vi "Pre Launch Init.vi"(11 "AsmTestMachine in":refnum<class "AsmTestMachine.lvclass">) -> (0 "error out":errorcluster, 3 "AsmTestMachine out":refnum<class "AsmTestMachine.lvclass">)   [LabVIEW 2021, in "AsmTestMachine.lvlib" / "AsmTestMachine.lvclass"]
doc: "(<B>Filename</B>: Actor Framework.lvlib:Actor.lvclass:Pre Launch Init.vi)\n\nDefines behavior that occurs after the Launch Nested Actor method is invoked but before the actor's Actor Core method begins running.\n\nBy default, this method does nothing. A descendant class may override it to define behavior."
uses:
  AsmTestMachine.lvclass
  Source/ActorStateMachine/ActorStateMachine/_ASM.State.ctl
  AsmTestMachine.lvclass/AsmTestMachine.ctl
  Source/ActorStateMachine/ActorStateMachine/ActorStateMachine.lvclass
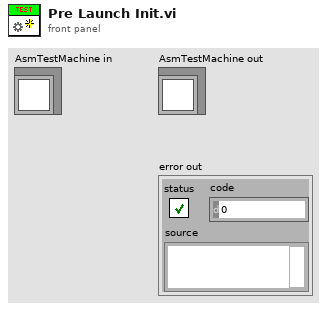
[diagram p1: front panel]
types:
  T1 = typedef "ActorStateMachine.lvlib/ActorStateMachine.lvclass/_ASM.State.ctl" = enum16{"Boom", "Pre-Init", "Init", "Post-Init", "Pre-Reset", "Reset", "Post-Reset", "Pre-Config", "Config", "Post-Config", "Pre-Ready", "Ready", "Post-Ready", "Pre-Running", "Running", "Next", "Post-Running", "Break", "Fail", "Crash", "Shutdown", "Doom"}
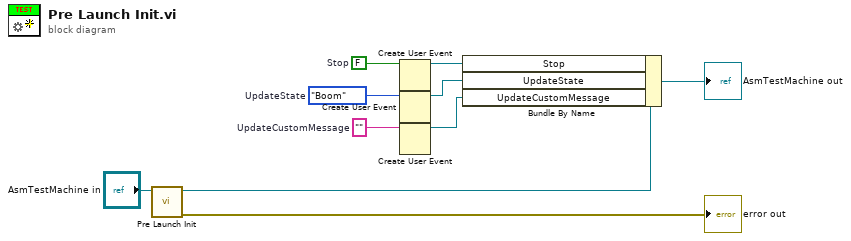
[diagram p0: block diagram]
diagram:
  w6 = ""  # UpdateCustomMessage
  w7 = _ASM.State."Boom"  # UpdateState
  w8 = FALSE  # Stop
  n1 = call-parent "Pre Launch Init.vi"("ActorStateMachine in"="AsmTestMachine in") -> ("error out"=→"error out":errorcluster, "ActorStateMachine out"=w5:refnum<class "AsmTestMachine.lvclass">)  [unwired: 9 in]
  n2 = Create User Event(user event datatype=w8) -> (user event=w3:refnum<user-event>)  [unwired: 1 in, 1 out]
  n3 = Create User Event(user event datatype=w7) -> (user event=w2:refnum<user-event>)  [unwired: 1 in, 1 out]
  n4 = Create User Event(user event datatype=w6) -> (user event=w1:refnum<user-event>)  [unwired: 1 in, 1 out]
  n5 = Bundle By Name(cluster=w5, "Stop"=w3, "UpdateState"=w2, "UpdateCustomMessage"=w1) -> (→"AsmTestMachine out":refnum<class "AsmTestMachine.lvclass">)
